vi "Test_fp_observer.vi"() -> ()   [LabVIEW 2017]
panel:
  in  "N_iters":i32
  out "Ax + Bu + Lye":sgl[](array[numeric])
  in  "X":sgl[](array[numeric])=[0.0, 0.0, 0.0, 0.0, 0.0, 0.0, 0.0, 0.0, 0.0, 0.0, 0.0, 0.0, 0.0, 0.0, 0.0, 0.0, 0.0, 0.0, 0.0, 0.0, 0.0, 0.0, 0.0, 0.0, 0.0]
  in  "u(k)":sgl format="%#_13g"
  in  "y(k)":sgl format="%#_13g"
  in  "NS":i16
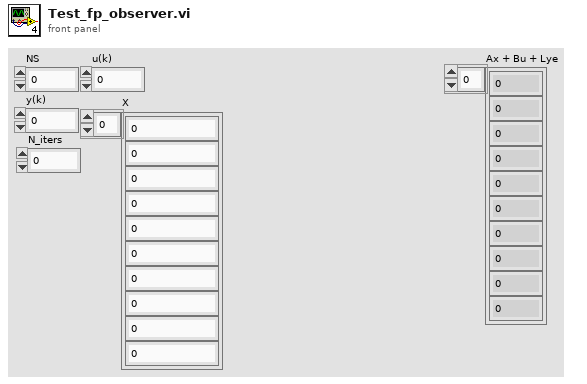
[diagram p1: front panel]
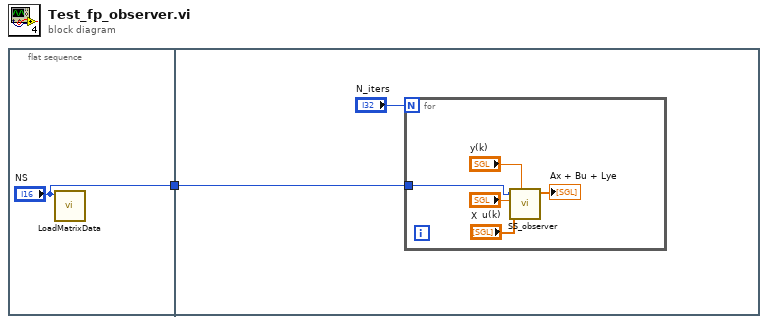
[diagram p0: block diagram]
diagram:
  n1 = flat-sequence {
    tunnel: ["NS"] -> w1
    tunnel: w1 -> [w4]
    frame #0 {
      n2 = call "LoadMatrixData.vi"("NS_control"="NS") -> ()  [unwired: 10 in, 1 out]
    }
    frame #1 {
      n3 = for {
        N: "N_iters" -> [_]
        tunnel: w4 -> [w8]
        n4 = call "SS_observer.vi"("y(k)"="y(k)", "X"="X", "u(k)"="u(k)", "NS"=w8) -> ("Ax + Bu + Lye"=→"Ax + Bu + Lye":sgl[])  [unwired: 7 in]
      }
    }
  }
